vi "Data Bank.vi"   [LabVIEW 2015]
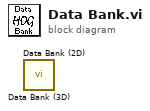
[diagram p0: block diagram]
diagram:
  n1 = call "Data Bank (3D).vi"() -> ()  [unwired: 13 in, 3 out]
  n2 = call "Data Bank (2D).vi"() -> ()  [unwired: 13 in, 3 out]
